vi "Signals.vi"() -> ()   [LabVIEW 2017]
panel:
  in  "Signals":string[][](array[string])
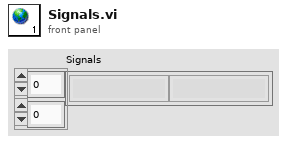
[diagram p1: front panel]
diagram:
